vi "RF_calibration_Keithley3390.vi"() -> ()   [LabVIEW 2017]
uses:
  instr.lib/Tektronix TDS 200 1000 2000 Series/Tektronix TDS 200 1000 2000 Series.lvlib
  <vilib>/Analysis/NI_AALPro.lvlib
  <vilib>/Analysis/6fits.llb/Curve Fitting Criteria.ctl
  instr.lib/Keithley 3390/Keithley 3390.lvlib
panel:
  out "Graph 2":cluster{dbl[], "Best Linear Fit":dbl[]}[](graph)=[{[120000.0, 121000.0, 122000.0, 123000.0, 124000.0, 125000.0, 126000.0, 127000.0, 128000.0, 129000.0, 130000.0, 131000.0, 132000.0, 133000.0, 134000.0, 135000.0, 136000.0, 137000.0, 138000.0, 139000.0], "Best Linear Fit"=[0.0, 0.0, 0.0, 0.0, 0.0, 0.0, 0.0, 0.0, 0.0, 0.0, 0.0, 0.0, 0.0, 0.0, 0.0, 0.0, 0.0, 0.0, 0.0, 0.0]}]
  out "Graph":cluster{dbl[], dbl[]}(graph)={[120000.0, 121000.0, 122000.0, 123000.0, 124000.0, 125000.0, 126000.0, 127000.0, 128000.0, 129000.0, 130000.0, 131000.0, 132000.0, 133000.0, 134000.0, 135000.0, 136000.0, 137000.0, 138000.0, 139000.0], [0.0, 0.0, 0.0, 0.0, 0.0, 0.0, 0.0, 0.0, 0.0, 0.0, 0.0, 0.0, 0.0, 0.0, 0.0, 0.0, 0.0, 0.0, 0.0, 0.0]}
  in  "Tab Control":enum32{"CONFIG", "MAIN", "DIAGNOSIS"}(tab)
  in  "Keithley3390":refnum<visa-resource-name>="USB0::0x05E6::0x3390::1269357::INSTR"
  in  "Columns":string[](array[string])=["FG freq (Hz)", "FG V (mVamp)", "Probe (1/100)(Vpp)", "Monitor (Vpp)"]
  in  "File path":path=path "C:/LabVIEW/DATA/J-PARC_202203/Filter_test"
  in  "Tektronix":refnum<visa-resource-name>="USB0::0x0699::0x0365::C035294::INSTR"
  out "File ref (calibration)":refnum<file>
  in  "COMMENT":string="test"
  in  "Tektronix test":bool
  in  "Refresh graph":bool
  out "current step":i32=19
  in  "sweep stop":bool
  in  "sweep start":bool
  in  "Tab Control 2":T1(tab)
  in  "f_start (Hz)":dbl=120000.0 format="%_8e"
  in  "f_end (Hz)":dbl=140000.0 format="%_8e"
  in  "ƒ¢f / cycle (Hz)":dbl=1000.0 format="%_8e"
  in  "V_start (mVamp)":dbl=1.0 format="%_6f"
  in  "V_end (mVamp)":dbl=10.0 format="%_6f"
  in  "ƒ¢V / cycle (mVamp)":dbl=1.0 format="%_6f"
  in  "freq/amp":bool
  in  "Vamp lower lim":dbl=0.4 format="%_4f"
  in  "Vamp upper lim":dbl=50.0 format="%_4f"
  in  "FG reset":bool
  in  "Amplitude (mVamp)":dbl=30.0 format="%_6f"
  in  "FG Output":bool
  in  "Frequency (Hz)":dbl=139000.0 format="%_8e"
  out "# of steps":i32=20
  out "Measurement index":i32=24
  out "Latest measurement":dbl[](array[numeric])=[139000.0, 30.0, 0.0, 0.0] format="%_8g"
  out "CH 1 measurement":dbl format="%_6g"
  out "CH 2 measurement":dbl format="%_6g"
  in  "Fit selecter":i32(ring) items=["No fitting", "Linear fit"]
  out "residue":dbl
  out "Fit results (slope, offset)":dbl[](array[numeric]) format="%_6e"
  out "error out (Agilent)":errorcluster
  out "error out (Tektronix)":errorcluster={"status"=TRUE, "code"=-1073807343, "source"="VISA Write in Tektronix_basic.vi->Tektronix_measure_2ch.vi->RF_calibration_Keithley3390.vi"}
  out "error out (file operation)":errorcluster
  in  "STOP":bool
  # "SWEEP SETTING"
  # "AGILENT CONTROL"
  # "Frequency sweep"
  # "Amplitude sweep"
  # "TEKTRONIX SETTING"
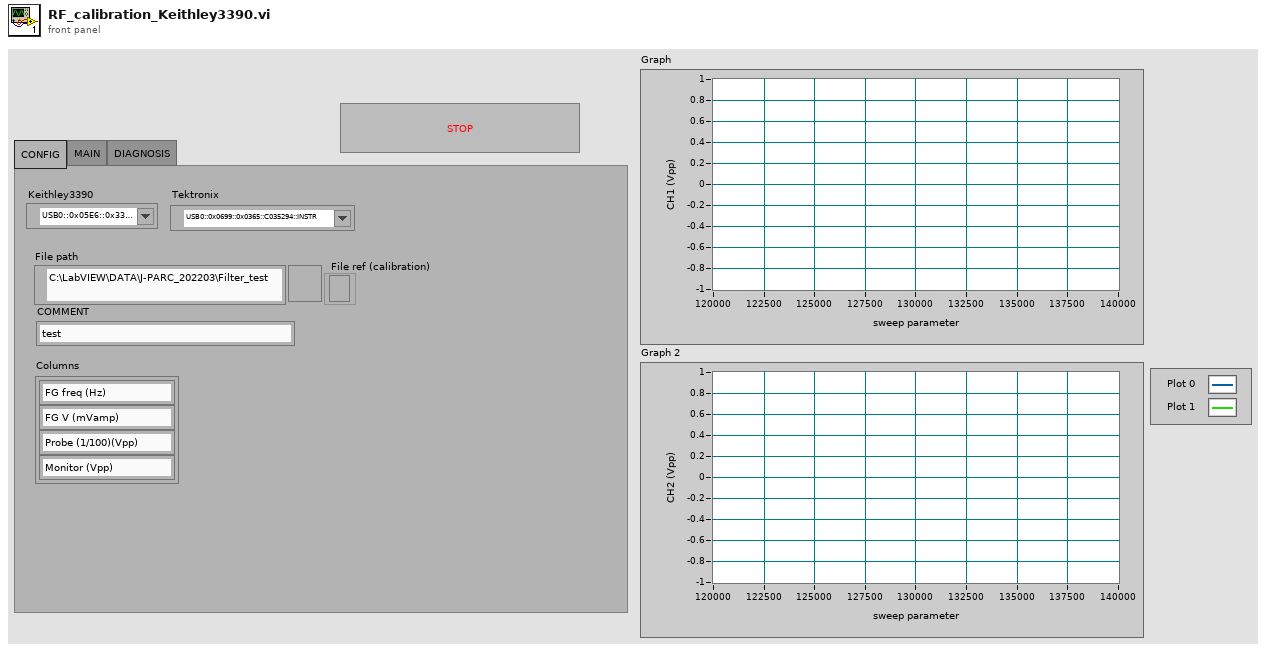
[diagram p1: front panel]
types:
  T1 = enum32{"frequency sweep config", "amplitude sweep config"}
  T2 = cluster{"Baud Rate":u32, "Parity":u16, "Stop Bits":u16, "Flow Control":u16}
  T3 = enum16{"open", "replace", "create", "open or create", "replace or create", "replace or create with confirmation"}
  T4 = cluster{"slope min":dbl, "slope max":dbl, "intercept min":dbl, "intercept max":dbl}
  T5 = typedef "NI_AALPro.lvlib/Curve Fitting Criteria.ctl" = u16
  T6 = cluster{"appended array":dbl[], "appended array":dbl[]}
  T7 = cluster{"appended array":dbl[], "appended array":dbl[]}[]
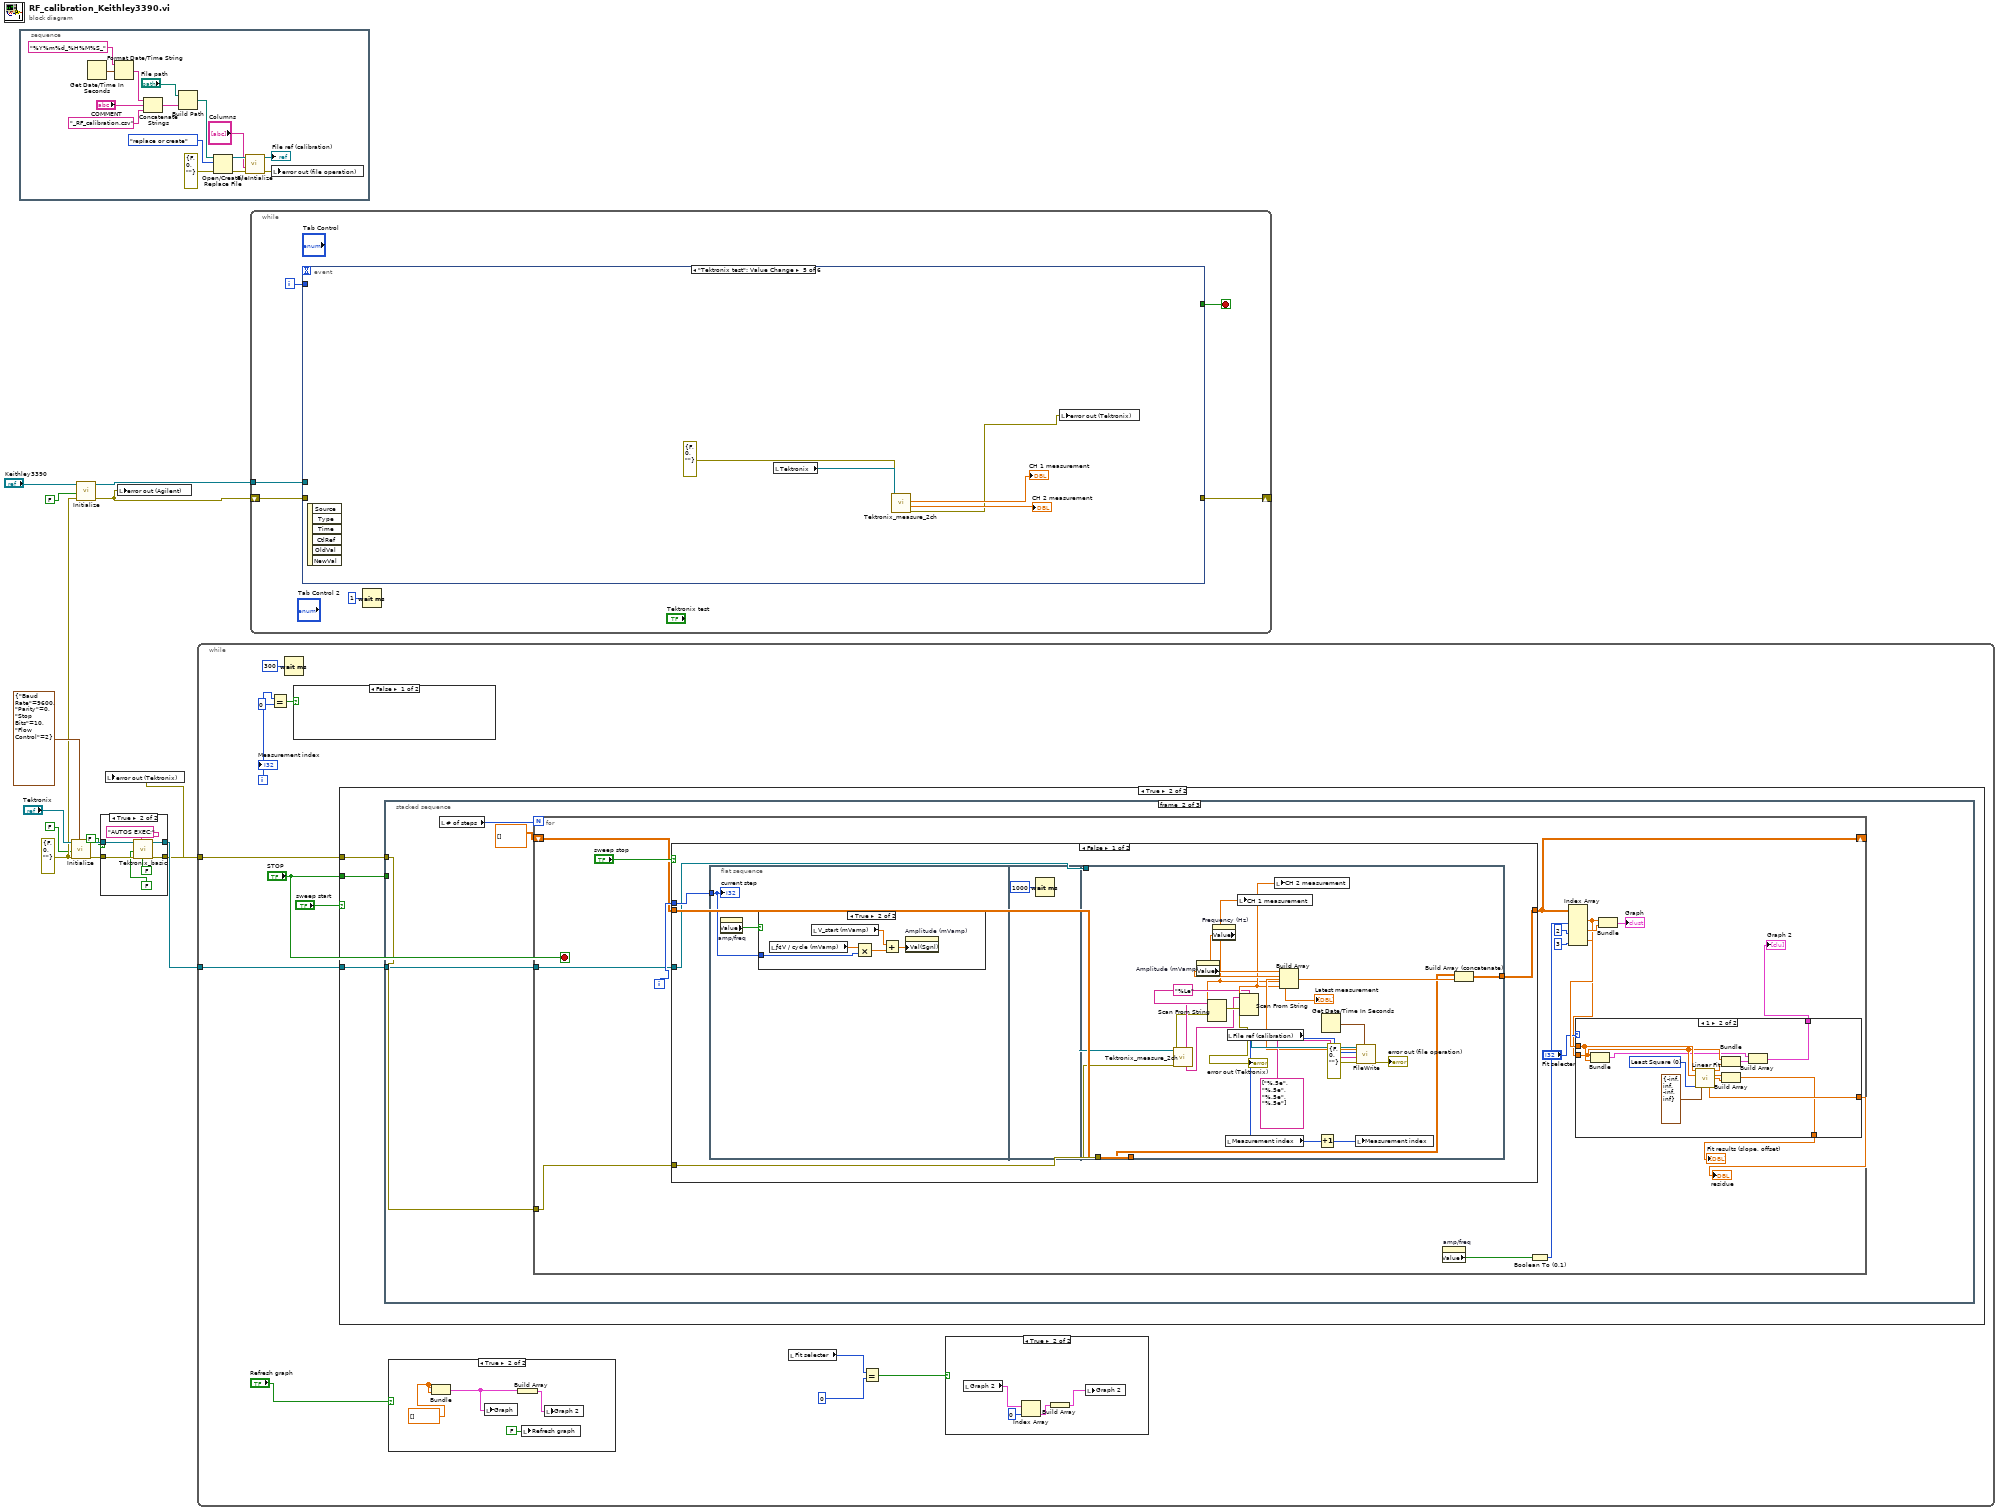
[diagram p0: block diagram]
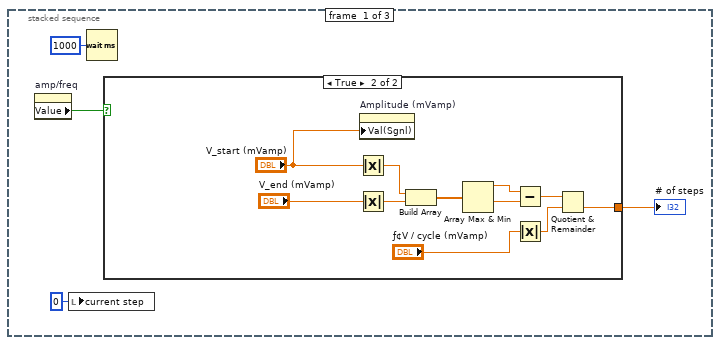
[diagram p6: hidden frame]
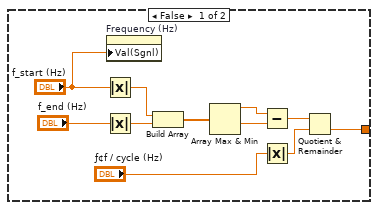
[diagram p7: hidden frame]
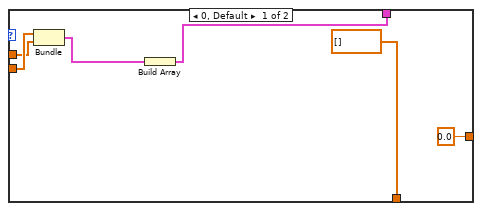
[diagram p8: hidden frame]
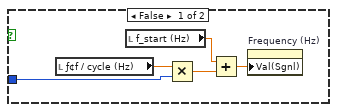
[diagram p9: hidden frame]
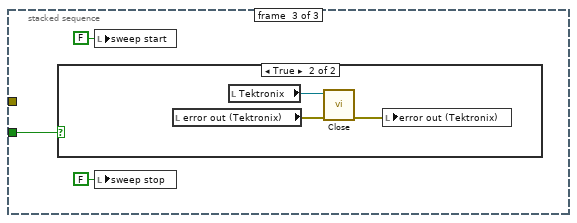
[diagram p11: hidden frame]
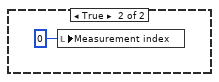
[diagram p13: hidden frame]
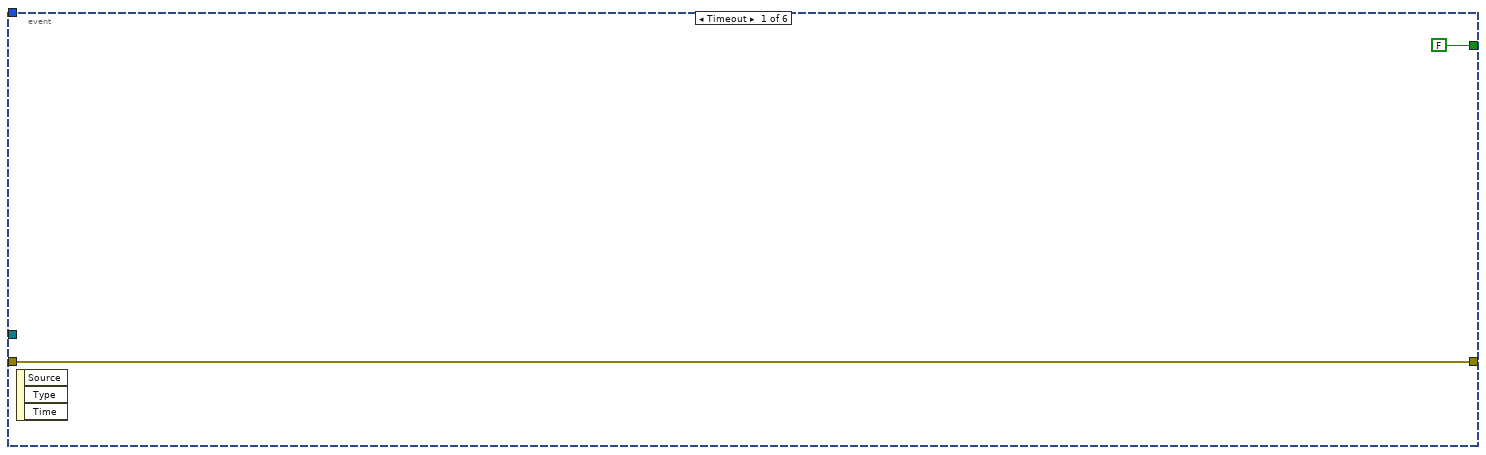
[diagram p14: hidden frame]
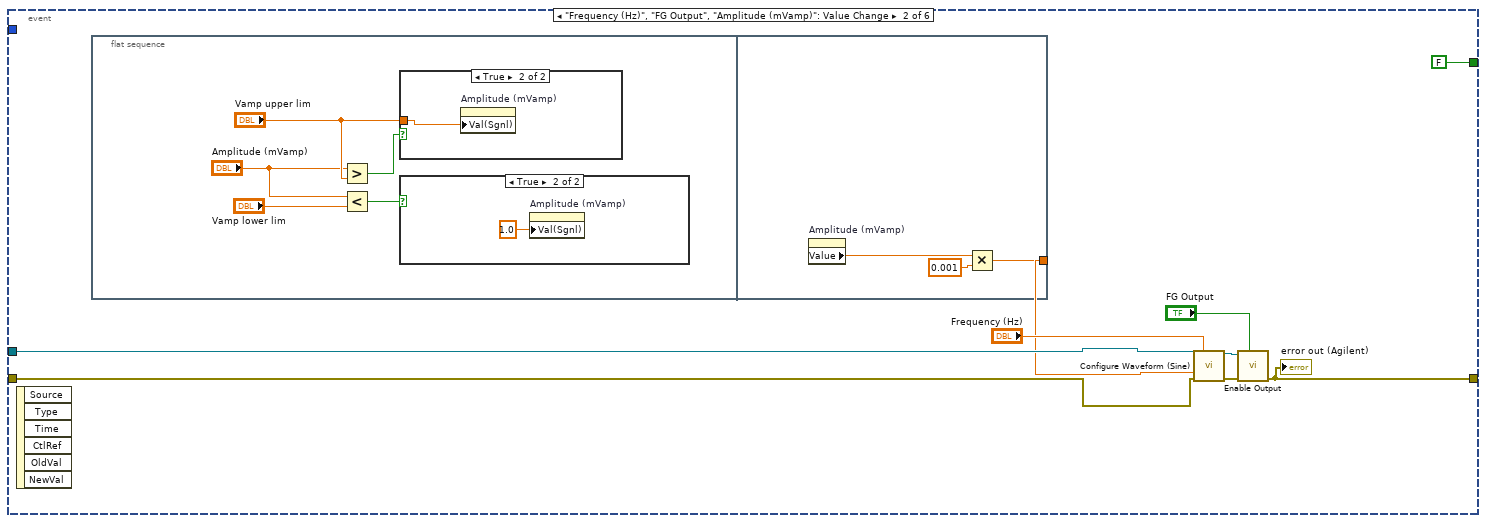
[diagram p15: hidden frame]
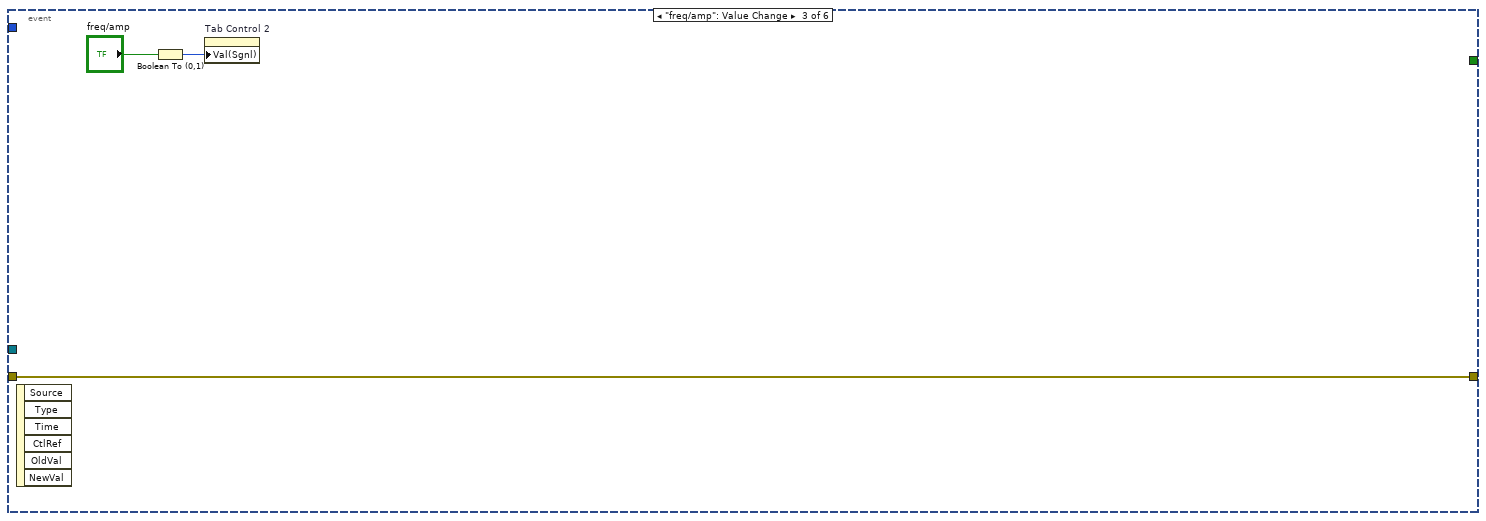
[diagram p18: hidden frame]
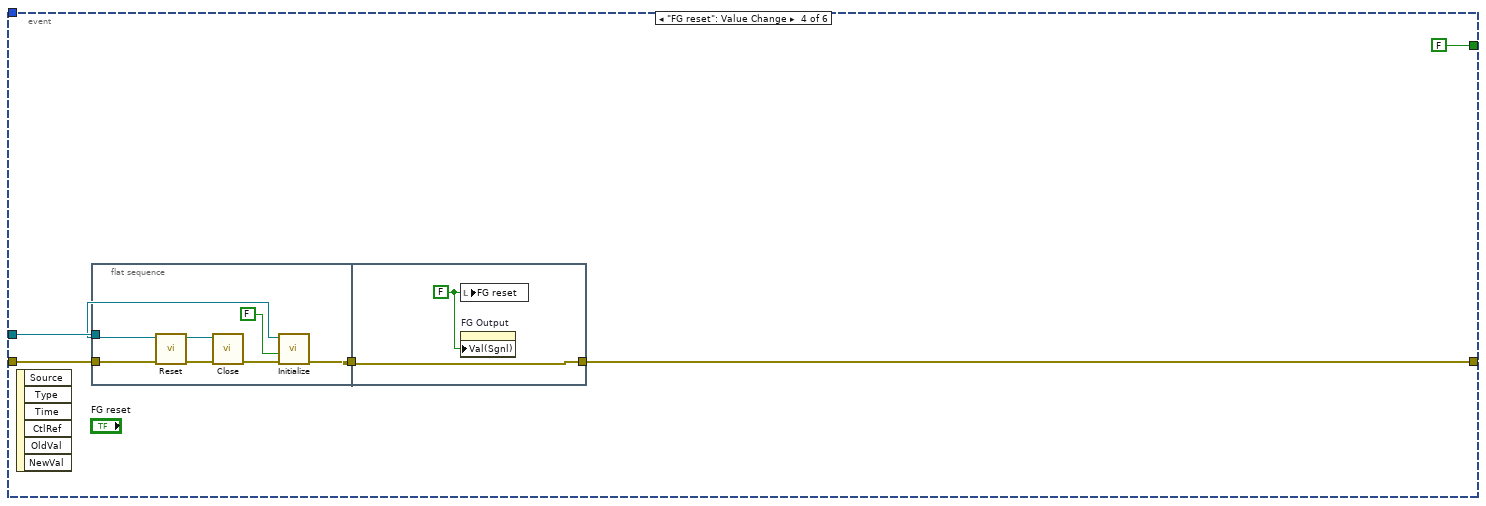
[diagram p19: hidden frame]
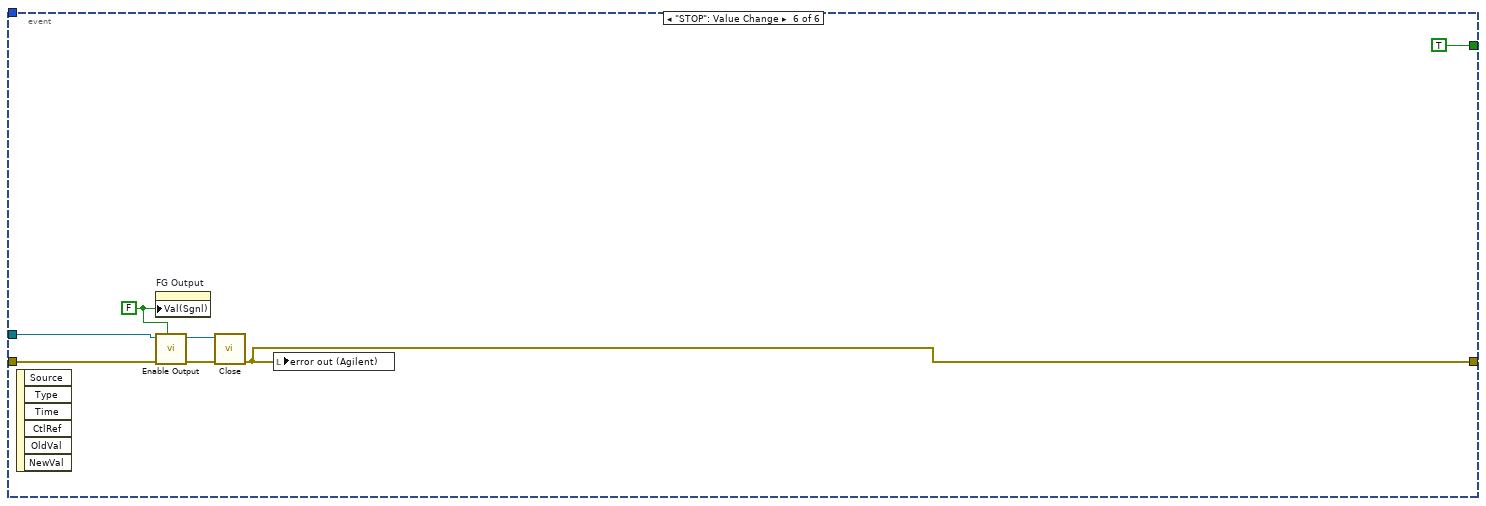
[diagram p20: hidden frame]
diagram:
  w7 = errorcluster {"status"=FALSE, "code"=0, "source"=""} ("error in (no error)")
  n1 = stacked-sequence {
    frame #0 {
      n2 = Get Date/Time In Seconds() -> (seconds since 1Jan1904=w17:timestamp)
      n3 = Format Date/Time String(time format string (%c)="%Y%m%d_%H%M%S_", seconds (now)=w17) -> (date/time string=w15:string)  [unwired: 1 in]
      n4 = Concatenate Strings(w15, "COMMENT", "_RF_calibration.csv") -> (w28:string)
      n5 = Build Path(base path="File path", name or relative path=w28) -> (appended path=w27:path)
      n6 = Open/Create/Replace File(file path (use dialog)=w27, error in=errorcluster {"status"=FALSE, "code"=0, "source"=""}, operation (0:open)=T3."replace or create") -> (refnum out=w24:refnum<file>, error out=w25:errorcluster)  [unwired: 3 in, 1 out]
      n7 = call "FileIntialize.vi"("Error In"=w25, "Labels"="Columns", "refnum in"=w24) -> ("Error Out"=w14:errorcluster, "File Refnum"=→"File ref (calibration)":refnum<file>)  [unwired: 7 in]
      n8 = local write "error out (file operation)"(w14) -> ()
    }
  }
  n9 = call "Initialize.vi"("Serial Configuration"=T2 {"Baud Rate"=9600, "Parity"=0, "Stop Bits"=10, "Flow Control"=2}, "error in (no error)"=w7, "Reset? (T: Yes)"=FALSE, "VISA resource name"="Tektronix") -> ("error out"=w5:errorcluster, "VISA resource name out"=w4:refnum<visa-resource-name>)  [unwired: 1 in, 5 out]
  n10 = call "Initialize.vi"("error in (no error)"=w7, "Reset (True)"=FALSE, "VISA resource name"="Keithley3390") -> ("error out"=w11:errorcluster, "VISA resource name out"=w12:refnum<visa-resource-name>)  [unwired: 7 in]
  n11 = case shown="True" FALSE {
    tunnel: w5 -> [w29 w37]
    tunnel: w4 -> [w30 w36]
    tunnel: [w30 w35] -> w3
    tunnel: [w29 w34] -> w2
    frame False {
    }
    frame True {
      n12 = call "Tektronix_basic.vi"("write buffer"="AUTOS EXEC;", "error in (no error)"=w37, "Query?"=FALSE, "Error query?"=FALSE, "VISA resource name"=w36) -> ("error out"=w34:errorcluster, "VISA resource name out"=w35:refnum<visa-resource-name>)  [unwired: 4 in, 1 out]
    }
  }
  n13 = local write "error out (Tektronix)"(w2) -> ()
  n14 = local write "error out (Agilent)"(w11) -> ()
  n15 = while {
    tunnel: w2 -> [w44]
    tunnel: w3 -> [w41]
    i -> [w49]
    stop <- "STOP" stop-if-true
    n16 = Equal?(x=w49, y=0) -> (x = y?=w47:bool)
    n17 = Wait (ms)(milliseconds to wait=u32 300) -> ()  [unwired: 1 out]
    n18 = case shown="False" w47 {
      frame False {
      }
      frame True {
        n19 = local write "Measurement index"(0 ("Measurement index")) -> ()
      }
    }
    n20 = case shown="True" "sweep start" {
      tunnel: w44 -> [_ w60]
      tunnel: "STOP" -> [_ w59]
      tunnel: w41 -> [_ w58]
      frame False {
      }
      frame True {
        n21 = stacked-sequence {
          tunnel: w60 -> [_ w90 _]
          tunnel: w59 -> [_ _ w170]
          tunnel: w58 -> [_ w87 _]
          frame #0 {
            n22 = property on="amp/freq" class="Bool (strict)"() -> ("Value"=w63:bool)  [unwired: 2 in, 2 out]
            n23 = local write "current step"(0 ("current step")) -> ()
            n24 = Wait (ms)(milliseconds to wait=u32 1000) -> ()  [unwired: 1 out]
            n25 = case shown="True" w63 {
              tunnel: [w65 w76] -> w64
              frame False {
                n26 = Absolute Value(x="f_start (Hz)") -> (abs(x)=w72:dbl)
                n27 = Absolute Value(x="f_end (Hz)") -> (abs(x)=w71:dbl)
                n28 = property on="Frequency (Hz)" class="DigNum (strict)"("Val(Sgnl)"="f_start (Hz)") -> ()  [unwired: 2 in, 2 out]
                n29 = Build Array(w72, w71) -> (w70:dbl[])
                n30 = Array Max & Min(array=w70) -> (max value=w69:dbl, min value=w68:dbl)  [unwired: 2 out]
                n31 = Subtract(x=w69, y=w68) -> (x-y=w67:dbl)
                n32 = Absolute Value(x="ƒ¢f / cycle (Hz)") -> (abs(x)=w74:dbl)
                n33 = Quotient & Remainder(x=w67, y=w74) -> (floor(x/y)=w65:dbl)  [unwired: 1 out]
              }
              frame True {
                n34 = Absolute Value(x="V_start (mVamp)") -> (abs(x)=w79:dbl)
                n35 = Absolute Value(x="V_end (mVamp)") -> (abs(x)=w80:dbl)
                n36 = property on="Amplitude (mVamp)" class="DigNum (strict)"("Val(Sgnl)"="V_start (mVamp)") -> ()  [unwired: 2 in, 2 out]
                n37 = Build Array(w79, w80) -> (w81:dbl[])
                n38 = Array Max & Min(array=w81) -> (max value=w82:dbl, min value=w83:dbl)  [unwired: 2 out]
                n39 = Subtract(x=w82, y=w83) -> (x-y=w84:dbl)
                n40 = Absolute Value(x="ƒ¢V / cycle (mVamp)") -> (abs(x)=w86:dbl)
                n41 = Quotient & Remainder(x=w84, y=w86) -> (floor(x/y)=w76:dbl)  [unwired: 1 out]
              }
            }
            "# of steps" <- w64
          }
          frame #1 {
            n42 = local read "# of steps"() -> (w89:i32)
            n43 = for {
              N: w89 -> [_]
              tunnel: w90 -> [w107]
              shift-right: [w104] -> _
              shift-left: dbl[][] [] -> [w105]
              tunnel: w87 -> [w97]
              i -> [w108]
              n44 = case shown="False" "sweep stop" {
                tunnel: w108 -> [w131 _]
                tunnel: w107 -> [w130 _]
                tunnel: [w129 w167] -> w104
                tunnel: w105 -> [w128 w167]
                tunnel: w97 -> [w127 _]
                frame False {
                  n45 = flat-sequence {
                    tunnel: w131 -> [w132]
                    tunnel: w130 -> [w163]
                    tunnel: [w156] -> w129
                    tunnel: w128 -> [w154]
                    tunnel: w127 -> [w153]
                    frame #0 {
                      n46 = property on="amp/freq" class="Bool (strict)"() -> ("Value"=w133:bool)  [unwired: 2 in, 2 out]
                      n47 = case shown="True" w133 {
                        tunnel: w132 -> [w136 w141]
                        frame False {
                          n48 = local read "ƒ¢f / cycle (Hz)"() -> (w137:dbl)
                          n49 = local read "f_start (Hz)"() -> (w138:dbl)
                          n50 = Multiply(x=w137, y=w136) -> (x*y=w135:dbl)
                          n51 = Add(x=w138, y=w135) -> (x+y=w134:dbl)
                          n52 = property on="Frequency (Hz)" class="DigNum (strict)"("Val(Sgnl)"=w134) -> ()  [unwired: 2 in, 2 out]
                        }
                        frame True {
                          n53 = local read "ƒ¢V / cycle (mVamp)"() -> (w142:dbl)
                          n54 = local read "V_start (mVamp)"() -> (w143:dbl)
                          n55 = Multiply(x=w142, y=w141) -> (x*y=w140:dbl)
                          n56 = Add(x=w143, y=w140) -> (x+y=w139:dbl)
                          n57 = property on="Amplitude (mVamp)" class="DigNum (strict)"("Val(Sgnl)"=w139) -> ()  [unwired: 2 in, 2 out]
                        }
                      }
                      "current step" <- w132
                    }
                    frame #1 {
                      n58 = Wait (ms)(milliseconds to wait=u32 1000) -> ()  [unwired: 1 out]
                    }
                    frame #2 {
                      w150 = "%Le" ("format string")
                      n59 = call "Tektronix_measure_2ch.vi"("error in (no error)"=w163, "VISA resource name"=w153) -> ("error out"=w146:errorcluster, "read buffer 2"=w149:string, "read buffer 1"=w148:string)  [unwired: 4 in, 3 out]
                      n60 = property on="Amplitude (mVamp)" class="DigNum (strict)"() -> ("Value"=w159:dbl)  [unwired: 2 in, 2 out]
                      n61 = Scan From String(format string=w150, input string=w148, error in=w146) -> (error out=w151:errorcluster, output 1=w147:dbl)  [unwired: 1 in, 3 out]
                      n62 = property on="Frequency (Hz)" class="DigNum (strict)"() -> ("Value"=w160:dbl)  [unwired: 2 in, 2 out]
                      n63 = local read "Measurement index"() -> (w157:i32)
                      n64 = local read "File ref (calibration)"() -> (w166:refnum<file>)
                      n65 = local write "CH 1 measurement"(w147) -> ()
                      n66 = Scan From String(format string=w150, input string=w149, error in=w151) -> (error out=→"error out (Tektronix)":errorcluster, output 1=w152:dbl)  [unwired: 1 in, 3 out]
                      n67 = local write "CH 2 measurement"(w152) -> ()
                      n68 = Build Array(w160, w159, w147, w152) -> (w155:dbl[])
                      "Latest measurement" <- w155
                      n69 = Increment(x=w157) -> (x+1=w158:i32)
                      n70 = Get Date/Time In Seconds() -> (seconds since 1Jan1904=w162:timestamp)
                      n71 = local write "Measurement index"(w158) -> ()
                      n72 = call "FileWrite.vi"("DataArray"=w155, "Time Stamp"=w162, "Error In"=errorcluster {"status"=FALSE, "code"=0, "source"=""}, "FileFormat"=string[] ["%.5e", "%.5e", "%.5e", "%.5e"], "Index"=w157, "refnum in"=w166) -> ("Error Out"=→"error out (file operation)":errorcluster)  [unwired: 4 in, 1 out]
                      n73 = Build Array (concatenate)(w154, w155) -> (w156:dbl[][])
                    }
                  }
                }
                frame True {
                }
              }
              n74 = property on="amp/freq" class="Bool (strict)"() -> ("Value"=w98:bool)  [unwired: 2 in, 2 out]
              n75 = Boolean To (0,1)(Boolean=w98) -> (0, 1=w101:i16)
              n76 = Index Array(array=w104, index (col) #1=w101, index (col) #2=2 ("disabled index (col)"), index (col) #3=3 ("index (row)")) -> (element #1=w92:dbl[], element #2=w103:dbl[], element #3=w96:dbl[])  [unwired: 3 in]
              n77 = case shown="1" "Fit selecter" {
                tunnel: w96 -> [w111 w119]
                tunnel: [0.0 ("residue") w122] -> w94
                tunnel: [dbl[] [] w121] -> w93
                tunnel: w92 -> [w112 w118]
                tunnel: [w109 w115] -> w91
                frame 0, Default {
                  n78 = Bundle(w112, w111) -> (w110:cluster{dbl[], dbl[]})  [unwired: 1 in]
                  n79 = Build Array(w110) -> (w109:cluster{dbl[], dbl[]}[])
                }
                frame 1 {
                  w126 = T5 0 items=["Least Square", "Least Absolute Residual", "Bisquare"] ("method")
                  n80 = Bundle(w118, w119) -> (w117:cluster{dbl[], dbl[]})  [unwired: 1 in]
                  n81 = call <vilib>:"Linear Fit.vi"("Y"=w119, "X"=w118, "method"=w126, "parameter bounds"=T4 {"slope min"=-inf, "slope max"=inf, "intercept min"=-inf, "intercept max"=inf}) -> ("Best Linear Fit"=w120:dbl[], "slope"=w124:dbl, "intercept"=w123:dbl, "residue"=w122:dbl)  [unwired: 7 in, 1 out]
                  n82 = Bundle(w118, "Best Linear Fit"=w120) -> (w116:cluster{dbl[], "Best Linear Fit":dbl[]})  [unwired: 1 in]
                  n83 = Build Array(w124, w123) -> (w121:dbl[])
                  n84 = Build Array(w117, w116) -> (w115:cluster{dbl[], "Best Linear Fit":dbl[]}[])
                }
              }
              "Graph 2" <- w91
              "residue" <- w94
              "Fit results (slope, offset)" <- w93
              n85 = Bundle(w92, w103) -> (→"Graph":cluster{dbl[], dbl[]})  [unwired: 1 in]
            }
          }
          frame #2 {
            n86 = case shown="True" w170 {
              frame False {
              }
              frame True {
                n87 = local read "error out (Tektronix)"() -> (w172:errorcluster)
                n88 = local read "Tektronix"() -> (w173:refnum<visa-resource-name>)
                n89 = call "Close.vi"("error in (no error)"=w172, "VISA resource name"=w173) -> ("error out"=w171:errorcluster)  [unwired: 9 out]
                n90 = local write "error out (Tektronix)"(w171) -> ()
              }
            }
            n91 = local write "sweep start"(FALSE ("sweep start")) -> ()
            n92 = local write "sweep stop"(FALSE ("sweep stop")) -> ()
          }
        }
      }
    }
    n93 = case shown="True" "Refresh graph" {
      frame False {
      }
      frame True {
        w57 = dbl[] [] ("appended array")
        n94 = Bundle("appended array"=w57, "appended array"=w57) -> (w55:T6)  [unwired: 1 in]
        n95 = local write "Graph"(w55) -> ()
        n96 = Build Array(w55) -> (w54:T7)
        n97 = local write "Refresh graph"(FALSE ("Refresh graph")) -> ()
        n98 = local write "Graph 2"(w54) -> ()
      }
    }
    n99 = local read "Fit selecter"() -> (w40:i32)
    n100 = Equal?(x=w40, y=0) -> (x = y?=w38:bool)
    n101 = case shown="True" w38 {
      frame False {
      }
      frame True {
        n102 = local read "Graph 2"() -> (w53:cluster{dbl[], "Best Linear Fit":dbl[]}[])
        n103 = Index Array(array=w53, index=0) -> (element=w51:cluster{dbl[], "Best Linear Fit":dbl[]})
        n104 = Build Array(w51) -> (w50:cluster{dbl[], "Best Linear Fit":dbl[]}[])
        n105 = local write "Graph 2"(w50) -> ()
      }
    }
  }
  n106 = while {
    tunnel: w12 -> [w180]
    shift-right: [w177] -> _
    shift-left: w11 -> [w176]
    i -> [w175]
    stop <- w178 stop-if-true
    n107 = event shown="[4] \"Tektronix test\": Value Change" {
      selector: _ -> [_ _ _ _ _ _]
      dyn-events: _ -> [_ _ _ _ _ _]
      timeout: _ -> [_ _ _ _ _ _]
      tunnel: w180 -> [_ w188 _ w207 _ w229]
      tunnel: w176 -> [w181 w187 w202 w205 _ w225]
      tunnel: [FALSE FALSE _ FALSE _ TRUE] -> w178
      tunnel: [w181 w186 w202 w209 _ w224] -> w177
      tunnel: w175 -> [_ _ _ _ _ _]
      event Timeout {
        n108 = event-data() -> ()  [unwired: 1 in, 3 out]
      }
      event "Frequency (Hz)", "FG Output", "Amplitude (mVamp)": Value Change {
        n109 = event-data() -> ()  [unwired: 1 in, 6 out]
        n110 = flat-sequence {
          tunnel: [w200] -> w184
          frame #0 {
            n111 = Greater?(x="Amplitude (mVamp)", y="Vamp upper lim") -> (0:w195:bool)
            n112 = Less?(x="Amplitude (mVamp)", y="Vamp lower lim") -> (x < y?=w192:bool)
            n113 = case shown="True" w195 {
              tunnel: "Vamp upper lim" -> [_ w198]
              frame False {
              }
              frame True {
                n114 = property on="Amplitude (mVamp)" class="DigNum (strict)"("Val(Sgnl)"=w198) -> ()  [unwired: 2 in, 2 out]
              }
            }
            n115 = case shown="True" w192 {
              frame False {
              }
              frame True {
                n116 = property on="Amplitude (mVamp)" class="DigNum (strict)"("Val(Sgnl)"=1.0 ("Value (Signaling)")) -> ()  [unwired: 2 in, 2 out]
              }
            }
          }
          frame #1 {
            n117 = property on="Amplitude (mVamp)" class="DigNum (strict)"() -> ("Value"=w199:dbl)  [unwired: 2 in, 2 out]
            n118 = Multiply(x=w199, y=0.001) -> (x*y=w200:dbl)
          }
        }
        n119 = call "Configure Waveform (Sine).vi"("VISA resource name"=w188, "Frequency (1000 Hz)"="Frequency (Hz)", "Amplitude (1.0 Vpp)"=w184, "error in (no error)"=w187) -> ("VISA resource name out"=w190:refnum<visa-resource-name>, "error out"=w191:errorcluster)  [unwired: 10 in]
        n120 = call "Enable Output.vi"("Enable Output (T: Enable)"="FG Output", "error in (no error)"=w191, "VISA resource name"=w190) -> ("error out"=w186:errorcluster)  [unwired: 7 in, 1 out]
        "error out (Agilent)" <- w186
      }
      event "freq/amp": Value Change {
        n121 = event-data() -> ()  [unwired: 1 in, 6 out]
        n122 = Boolean To (0,1)(Boolean="freq/amp") -> (0, 1=w203:i16)
        n123 = property on="Tab Control 2" class="TabCtl (strict)"("Val(Sgnl)"=w203) -> ()  [unwired: 2 in, 2 out]
      }
      event "FG reset": Value Change {
        n124 = event-data() -> ()  [unwired: 1 in, 6 out]
        n125 = flat-sequence {
          tunnel: [w216] -> w206
          tunnel: w205 -> [w210]
          tunnel: w207 -> [w213]
          tunnel: [w218] -> w209
          tunnel: w206 -> [w218]
          frame #0 {
            n126 = call "Reset.vi"("error in (no error)"=w210, "VISA resource name"=w213) -> ("error out"=w211:errorcluster, "VISA resource name out"=w212:refnum<visa-resource-name>)  [unwired: 8 in]
            n127 = call "Close.vi"("error in (no error)"=w211, "VISA resource name"=w212) -> ("error out"=w215:errorcluster)  [unwired: 9 in]
            n128 = call "Initialize.vi"("error in (no error)"=w215, "Reset (True)"=FALSE ("ID Query (True)"), "VISA resource name"=w213) -> ("error out"=w216:errorcluster)  [unwired: 7 in, 1 out]
          }
          frame #1 {
            w217 = FALSE ("Value (Signaling)")
            n129 = local write "FG reset"(w217) -> ()
            n130 = property on="FG Output" class="Bool (strict)"("Val(Sgnl)"=w217) -> ()  [unwired: 2 in, 2 out]
          }
        }
      }
      event "Tektronix test": Value Change {
        n131 = event-data() -> ()  [unwired: 1 in, 6 out]
        n132 = local read "Tektronix"() -> (w223:refnum<visa-resource-name>)
        n133 = call "Tektronix_measure_2ch.vi"("error in (no error)"=errorcluster {"status"=FALSE, "code"=0, "source"=""}, "VISA resource name"=w223) -> ("error out"=w219:errorcluster, "Measurement 2"=→"CH 2 measurement":dbl, "Measurement 1"=→"CH 1 measurement":dbl)  [unwired: 4 in, 3 out]
        n134 = local write "error out (Tektronix)"(w219) -> ()
      }
      event "STOP": Value Change {
        w227 = FALSE ("Enable Output  (T: Enable)")
        n135 = event-data() -> ()  [unwired: 1 in, 6 out]
        n136 = property on="FG Output" class="Bool (strict)"("Val(Sgnl)"=w227) -> ()  [unwired: 2 in, 2 out]
        n137 = call "Enable Output.vi"("Enable Output (T: Enable)"=w227, "error in (no error)"=w225, "VISA resource name"=w229) -> ("error out"=w228:errorcluster, "VISA resource name out"=w230:refnum<visa-resource-name>)  [unwired: 7 in]
        n138 = call "Close.vi"("error in (no error)"=w228, "VISA resource name"=w230) -> ("error out"=w224:errorcluster)  [unwired: 9 in]
        n139 = local write "error out (Agilent)"(w224) -> ()
      }
    }
    n140 = Wait (ms)(milliseconds to wait=u32 1) -> ()  [unwired: 1 out]
  }
